vi "Operation.vi"(0 "Subtract in":refnum<class "Subtract.lvclass">, 11 "Error In":errorcluster) -> (4 "Subtract out":refnum<class "Subtract.lvclass">, 15 "Error Out":errorcluster)   [LabVIEW 2020, in "Subtract.lvclass"]
doc: "Method to perform the division operation."
uses:
  Subtract.lvclass
  Subtract.lvclass/Subtract.ctl
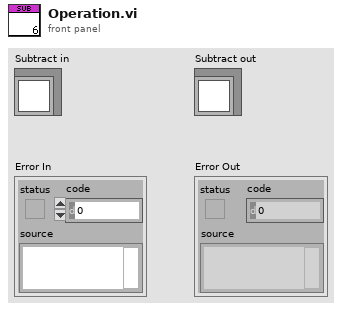
[diagram p1: front panel]
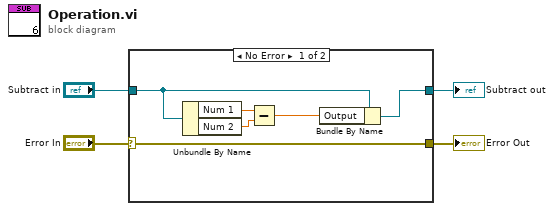
[diagram p0: block diagram]
diagram:
  n1 = case shown="No Error" "Error In" {
    selector: "Error In" -> [w10 w12]
    tunnel: [w10 w12] -> w3
    tunnel: [w6 w11] -> w1
    tunnel: "Subtract in" -> [w9 w11]
    frame No Error {
      n2 = Unbundle By Name(w9) -> ("Num 1"=w7:dbl, "Num 2"=w8:dbl)
      n3 = Subtract(x=w7, y=w8) -> (x-y=w5:dbl)
      n4 = Bundle By Name(cluster=w9, "Output"=w5) -> (w6:refnum<class "Subtract.lvclass">)
    }
    frame Error {
    }
  }
  "Error Out" <- w3
  "Subtract out" <- w1
